vi "Med_Fases.vi"() -> (6 "TENSÃO FASE A":dynamicdata(graph))   [LabVIEW 2025]
panel:
  out "TENSÃO / CORRENTE FASE C":string[][](table)
  out "CORRENTE FASE C":dynamicdata(graph)
  out "TENSÃO FASE C":dynamicdata(graph)
  out "TENSÃO / CORRENTE FASE B":string[][](table)
  out "CORRENTE FASE B":dynamicdata(graph)
  out "TENSÃO FASE B":dynamicdata(graph)
  out "TENSÃO / CORRENTE FASE A":string[][](table)
  out "CORRENTE FASE A":dynamicdata(graph)
  out "Table 2":string[][](table)
  out "Table":string[][](table)
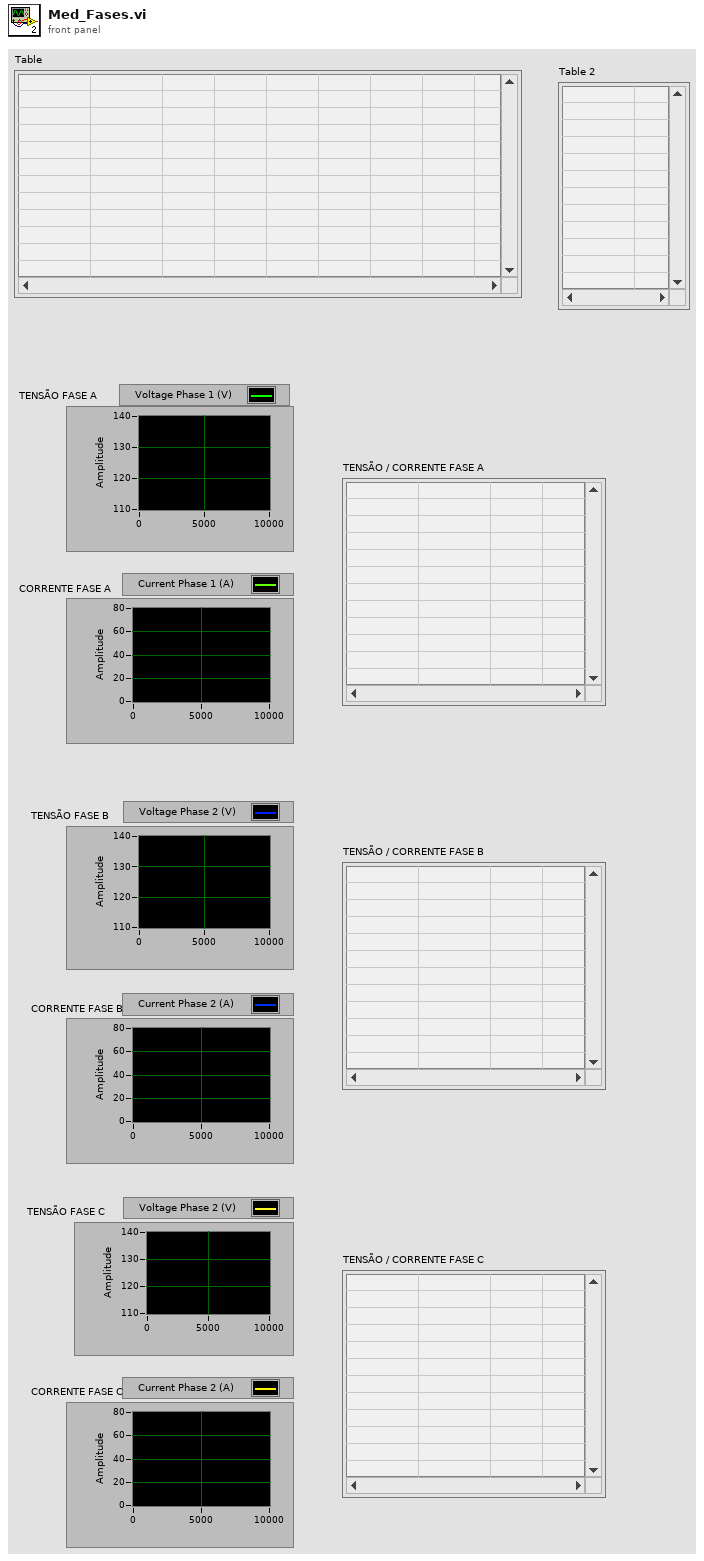
[diagram p1: front panel]
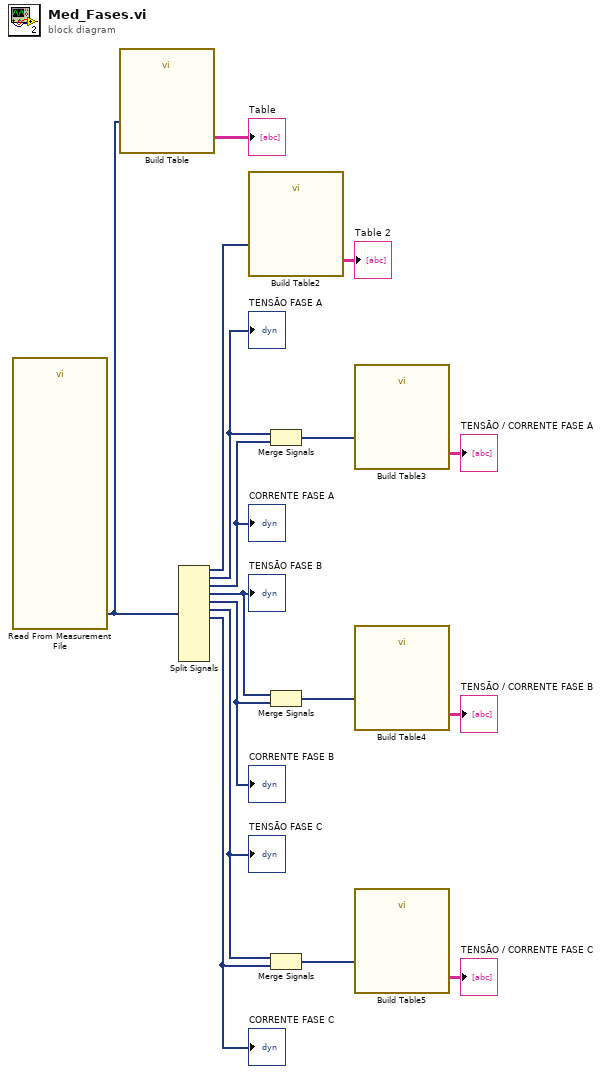
[diagram p0: block diagram]
diagram:
  n1 = call "Read From Measurement File"() -> ("Signals"=w15:dynamicdata)  [unwired: 6 in, 5 out]
  n2 = call "Build Table"("Signals"=w15) -> ("Table"=→"Table":string[][])  [unwired: 4 in, 6 out]
  n3 = Split Signals(w15) -> (w13:dynamicdata, w12:dynamicdata, w11:dynamicdata, w6:dynamicdata, w5:dynamicdata, w2:dynamicdata, w1:dynamicdata)  [unwired: 12 in, 5 out]
  "TENSÃO FASE A" <- w12
  "CORRENTE FASE A" <- w11
  "TENSÃO FASE B" <- w6
  "CORRENTE FASE B" <- w5
  "TENSÃO FASE C" <- w2
  "CORRENTE FASE C" <- w1
  n4 = call "Build Table2"("Signals"=w13) -> ("Table"=→"Table 2":string[][])  [unwired: 4 in, 6 out]
  n5 = Merge Signals(w12, w11) -> (w10:dynamicdata)
  n6 = Merge Signals(w6, w5) -> (w8:dynamicdata)
  n7 = Merge Signals(w2, w1) -> (w4:dynamicdata)
  n8 = call "Build Table3"("Signals"=w10) -> ("Table"=→"TENSÃO / CORRENTE FASE A":string[][])  [unwired: 4 in, 6 out]
  n9 = call "Build Table4"("Signals"=w8) -> ("Table"=→"TENSÃO / CORRENTE FASE B":string[][])  [unwired: 4 in, 6 out]
  n10 = call "Build Table5"("Signals"=w4) -> ("Table"=→"TENSÃO / CORRENTE FASE C":string[][])  [unwired: 4 in, 6 out]
